vi "CheckCollision.vi"(8 "error in":errorcluster, 10 "sprite in":refnum<class "Sprite.lvclass">, 11 "class data in":refnum<class "BoundingBox.lvclass">) -> (0 "error out":errorcluster, 1 "collisionInfo out":cluster{"collision":bool, "fatal":bool}, 2 "sprite out":refnum<class "Sprite.lvclass">, 3 "class data out":refnum<class "BoundingBox.lvclass">)   [LabVIEW 2010, in "Labricks.lvlib" / "BoundingBox.lvclass"]
uses:
  BoundingBox.lvclass
  RenderBase/Sprite_class/Sprite.lvclass
  BoundingBox.lvclass/BoundingBox.ctl
  RenderBase/SceneObject_class/properties/Position/GetPosition.vi
  RenderBase/Sprite_class/properties/Direction/GetDirection.vi
  Game_class/Game.lvclass
  RenderBase/SceneObject_class/SceneObject.lvclass
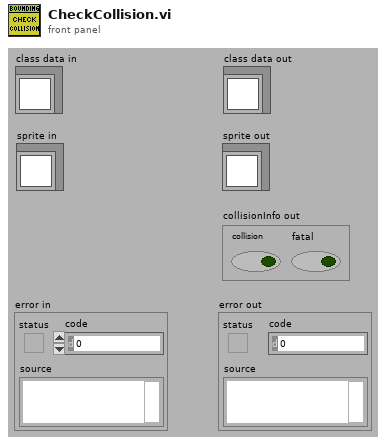
[diagram p1: front panel]
types:
  T1 = typedef "LV3DPointTypeDef.ctl" = cluster{"X":sgl, "Y":sgl, "Z":sgl}
  T2 = typedef "RenderBase.lvlib/SceneObject.lvclass/CollisionAction.ctl" = enum16{"None", "BounceX", "BounceY", "BounceXY"}
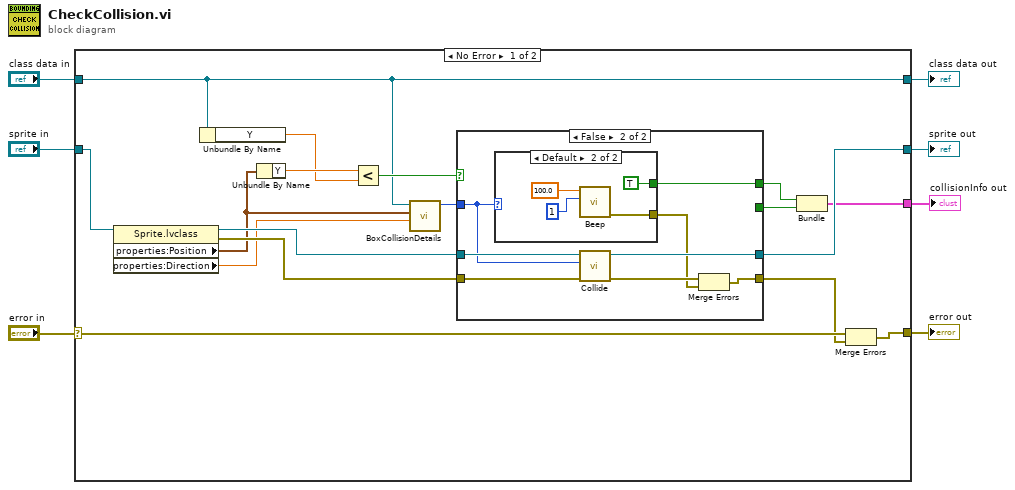
[diagram p0: block diagram]
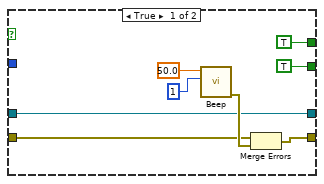
[diagram p2: hidden frame]
diagram:
  n1 = case shown="No Error" "error in" {
    selector: "error in" -> [w22 w47]
    tunnel: [w23 w47] -> w7
    tunnel: "sprite in" -> [w24 w45]
    tunnel: [w11 w46] -> w5
    tunnel: "class data in" -> [w11 w46]
    tunnel: [w21 w45] -> w2
    tunnel: [w18 _] -> w1
    frame No Error {
      n2 = property class="Sprite.lvclass"(reference=w24) -> (reference out=w17:refnum<class "Sprite.lvclass">, error out=w16:errorcluster, "properties:Position"=w10:T1, "properties:Direction"=w9:csg)  [unwired: 1 in]
      n3 = Unbundle By Name(w11) -> ("Y"=w14:sgl)
      n4 = Unbundle By Name(w10) -> ("Y"=w15:sgl)
      n5 = Less?(x=w15, y=w14) -> (x < y?=w13:bool)
      n6 = call "BoxCollisionDetails.vi"("direction in"=w9, "position in"=w10, "class data in"=w11) -> ("collisionAction out"=w8:T2)  [unwired: 8 in]
      n7 = case shown="False" w13 {
        tunnel: w17 -> [w27 w40]
        tunnel: [w27 w39] -> w21
        tunnel: [TRUE _] -> w19
        tunnel: w16 -> [w26 w38]
        tunnel: [w29 w36] -> w20
        tunnel: [TRUE w34] -> w12
        tunnel: w8 -> [_ w33]
        frame True {
          n8 = call "Beep.vi"("numChunks in"=1 ("#s"), "frequency in"=50.0 ("frequency")) -> ("error out"=w28:errorcluster)  [unwired: 9 in]
          n9 = Merge Errors(w26, w28) -> (w29:errorcluster)
        }
        frame False {
          n10 = case shown="Default" w33 {
            tunnel: [_ w42] -> w35
            tunnel: [_ TRUE] -> w34
            frame "None" {
            }
            frame Default {
              n11 = call "Beep.vi"("numChunks in"=1 ("#s"), "frequency in"=100.0 ("frequency")) -> ("error out"=w42:errorcluster)  [unwired: 9 in]
            }
          }
          n12 = call-dynamic "Collide.vi"("error in (no error)"=w38, "action in"=w33, "class data in"=w40) -> ("error out"=w37:errorcluster, "class data out"=w39:refnum<class "Sprite.lvclass">)  [unwired: 7 in]
          n13 = Merge Errors(w37, w35) -> (w36:errorcluster)
        }
      }
      n14 = Bundle(w12, w19) -> (w18:cluster{bool, bool})  [unwired: 1 in]
      n15 = Merge Errors(w22, w20) -> (w23:errorcluster)
    }
    frame Error {
    }
  }
  "error out" <- w7
  "class data out" <- w5
  "sprite out" <- w2
  "collisionInfo out" <- w1
